vi "Cluster.vi"() -> ()   [LabVIEW 2021]
panel:
  out "gender":bool
  out "salary":u16
  out "age 2":u8
  out "name":string
  in  "employee":T1
  in  "age":u8
  out "IndEmp":T1
  in  "employee":T1
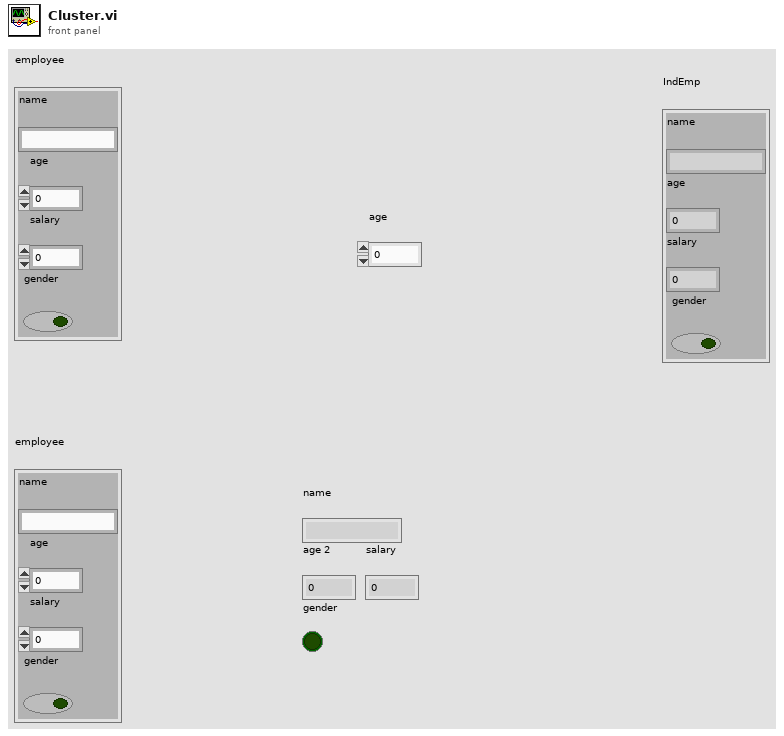
[diagram p1: front panel]
types:
  T1 = cluster{"name":string, "age":u8, "salary":u16, "gender":bool}
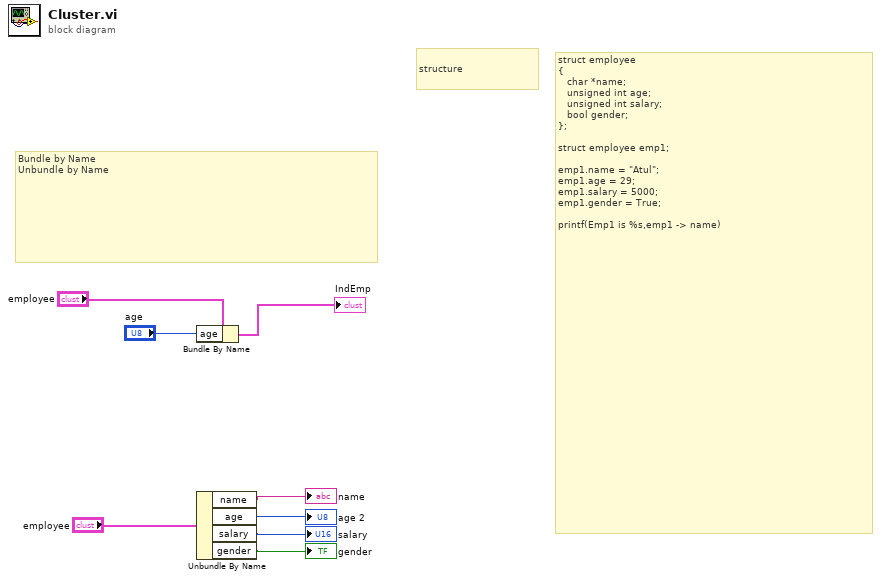
[diagram p0: block diagram]
diagram:
  # "Bundle by Name\nUnbundle by Name"
  # "struct employee\n{\n   char *name;\n   unsigned int age;\n   unsigned int salary;\n   bool gender;\n};\n\nstruct employee emp1;\n\nemp1.name = \"Atul\";\nemp1.age = 29;\nemp1.salary = 5000;\nemp1.gender = True;\n\nprintf(Emp1 is %s,emp1 -> name)"
  # "structure"
  n1 = Bundle By Name(cluster="employee", "age"="age") -> (→"IndEmp":T1)
  n2 = Unbundle By Name("employee") -> ("name"=→"name":string, "age"=→"age 2":u8, "salary"=→"salary":u16, "gender"=→"gender":bool)
